vi "Compute N-Exp Fit Optimal Offset.vi"(7 "Fit Control Data in":T8, 8 "Error In":errorcluster, 9 "Offset Array":dbl[](array[numeric]), 11 "Fit Output in":T1[](array[typedef])) -> (0 "Error Out":errorcluster, 1 "C_00":dbl, 3 "Fit Output out":T1={"best nonlinear fit"=[], "best fit parameters"=[], "R^2"=0.0, "RMSE"=0.0, "error out"={"status"=FALSE, "code"=0, "source"=""}, "Fitting Method"=enum."Least Square", "number of function calls"=0, "number of iterations"=0, "covariance"=[], "Chi 2"=0.0, "DOF"=0, "Fit Convergence Criterion"=enum."Continue", "Fitting Algorithm"=enum."Levenberg-Marquardt", "Weighted Fit"=enum."Unweighted", "Gradient"=0.0, "|Delta Chi 2|"=0.0, "|Delta Chi 2|/Chi 2"=0.0, "Max |Delta a| /|a|"=0.0, "Lambda"=-1.0, "RSS"=0.0, "AIC"=0.0, "BIC"=0.0, "Max number of function calls"=0, "Max number of iterations"=0, "IRF"={"X Array"=[], "Y Array"=[]}, "IRF Normalization Factor"=0.0, "Decay Normalization Factor"=0.0, "Number of offset fits"=0, "Weighted Chi2"=-1.0, "Unweighted Chi2"=-1.0}, 5 "Fit Control Data out":T8)   [LabVIEW 2021, in "Fits.lvlib"]
doc: "If more than 2 offsets have been tried, fits a parabola through the Chi^2 values to find the minimum location. and returns the curvatue C_00 used to computed the offset uncertainty.\nOtherwise, use the result with the smallest Chi^2."
uses:
  Fits.lvlib
  Non-linear Fit Output v4.ctl
  Nonlinear Fit Method.ctl
  <vilib>/Analysis/Matrix/Datatypes/RealMatrix.ctl
  Convergence Criteria.ctl
  Non-linear Fitting Algorithm.ctl
  IRF(X)PSED/Fit Weights Type v2.ctl
  Graphs/XY Graph/XY Graph Plot Data.ctl
  Decay Convolution/Fit Control Data v2.ctl
  IRF(X)PSED/Decay Fit Parameters In List.ctl
  Decay Convolution/Decay Model.ctl
  <vilib>/Analysis/Matrix/NI_Matrix.lvlib
  Graphs/XY Graph/XY Graph Add-Ons.lvlib
panel:
  out "~t_0":dbl
  out "Chi^2":dbl
  out "t_0":dbl
  out "XY Graph":T11(graph)
  # "see the AlliGator License on the block diagram (Ctrl+E or Window:Show Block Diagram)"
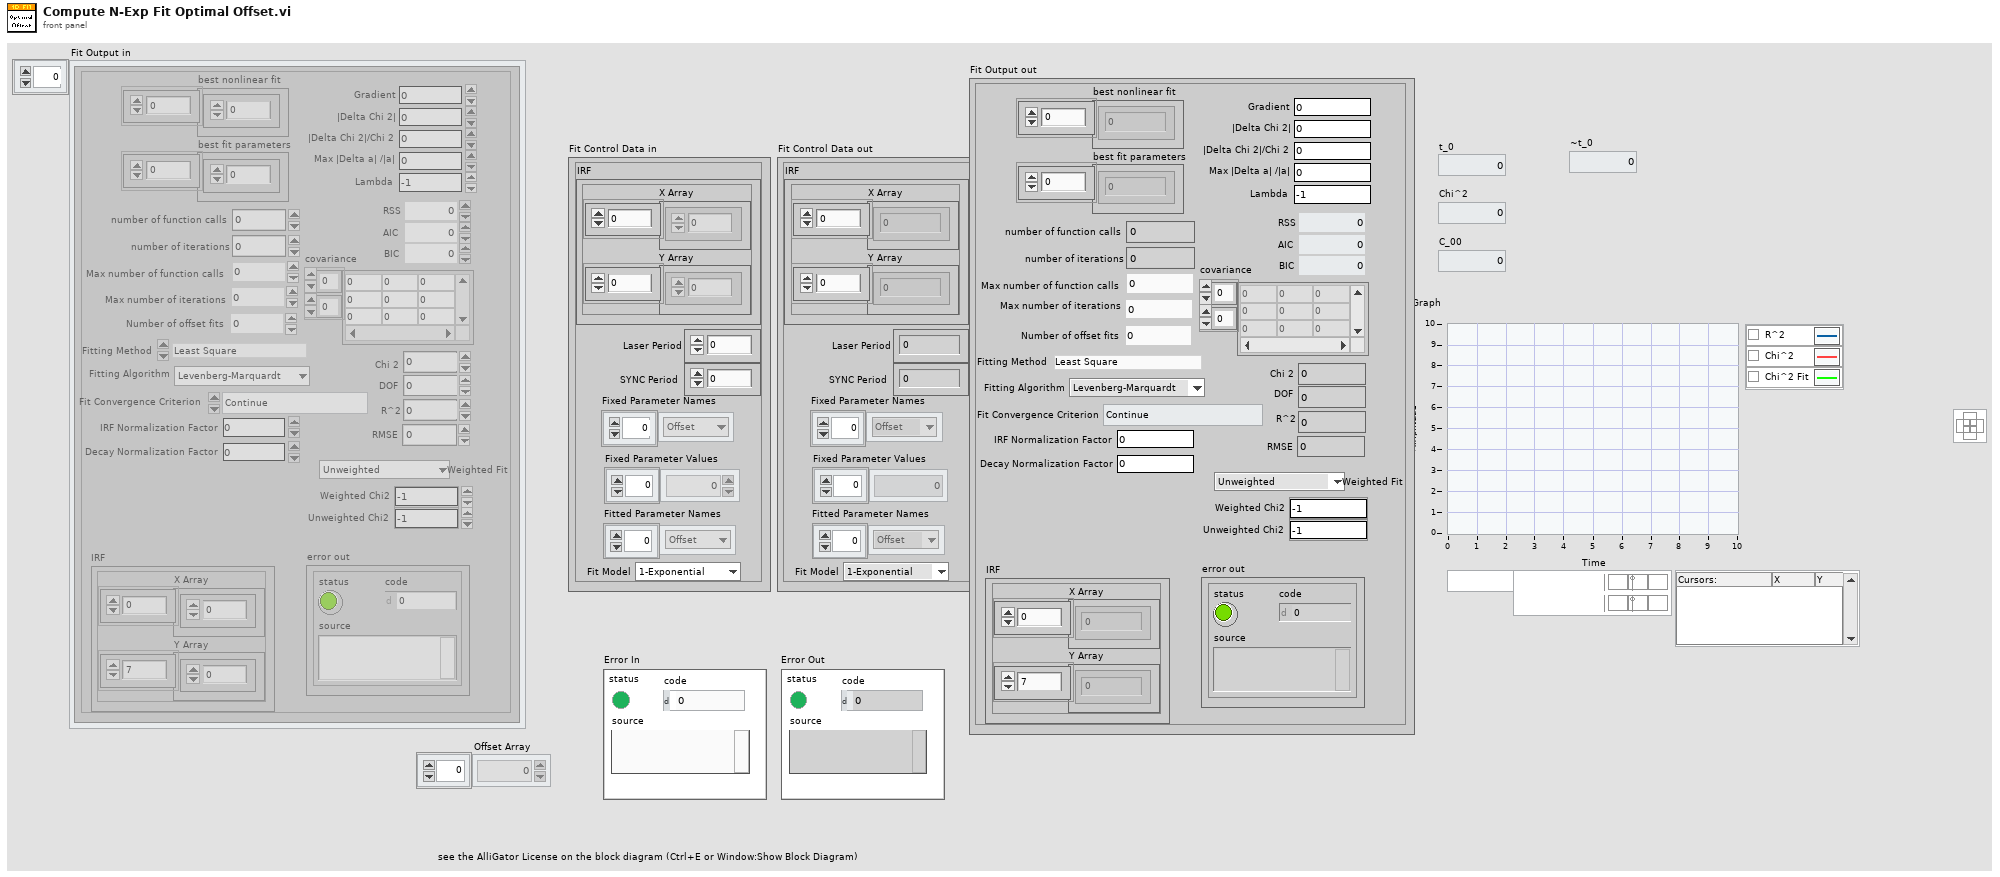
[diagram p1: front panel]
types:
  T1 = typedef "Fits.lvlib/Non-linear Fit Output v4.ctl" = cluster{"best nonlinear fit":dbl[], "best fit parameters":dbl[], "R^2":dbl, "RMSE":dbl, "error out":errorcluster, "Fitting Method":T2, "number of function calls":i32, "number of iterations":i32, "covariance":T3, "Chi 2":dbl, "DOF":i32, "Fit Convergence Criterion":T4, "Fitting Algorithm":T5, "Weighted Fit":T6, "Gradient":dbl, "|Delta Chi 2|":dbl, "|Delta Chi 2|/Chi 2":dbl, "Max |Delta a| /|a|":dbl, "Lambda":dbl, "RSS":dbl, "AIC":dbl, "BIC":dbl, "Max number of function calls":i32, "Max number of iterations":i32, "IRF":T7, "IRF Normalization Factor":dbl, "Decay Normalization Factor":dbl, "Number of offset fits":i32, "Weighted Chi2":dbl, "Unweighted Chi2":dbl}
  T2 = typedef "Fits.lvlib/Nonlinear Fit Method.ctl" = enum16{"Least Square", "Least Absolute Residual", "Bisquare", "MLE"}
  T3 = typedef "NI_Matrix.lvlib/RealMatrix.ctl" = dbl[][]
  T4 = typedef "Fits.lvlib/Convergence Criteria.ctl" = enum16{"Continue", "Tolerances Exceeded", "Max Time Exceeded", "Max Iterations Exceeded", "Max Function Evaluations Exceeded", "Scale Range Exceeded"}
  T5 = typedef "Fits.lvlib/Non-linear Fitting Algorithm.ctl" = enum16{"Levenberg-Marquardt", "Trust-Region Dogleg"}
  T6 = typedef "Fits.lvlib/Fit Weights Type v2.ctl" = enum16{"Unweighted", "1/Variance (Neyman)", "1/Variance (Pearson)", "Best of All"}
  T7 = typedef "XY Graph Add-Ons.lvlib/XY Graph Plot Data.ctl" = cluster{"X Array":dbl[], "Y Array":dbl[]}
  T8 = typedef "Fits.lvlib/Fit Control Data v2.ctl" = cluster{"IRF":T7, "Laser Period":dbl, "SYNC Period":dbl, "Fixed Parameter Names":T9[], "Fixed Parameter Values":dbl[], "Fitted Parameter Names":T9[], "Fit Model":T10}
  T9 = typedef "Fits.lvlib/Decay Fit Parameters In List.ctl" = enum16{"Offset", "Baseline", "A_1", "tau_1", "A_2", "tau_2"}
  T10 = typedef "Fits.lvlib/Decay Model.ctl" = enum16{"1-Exponential", "2-Exponentials"}
  T11 = cluster{"Offset Array":dbl[], "Best Polynomial Fit":dbl[]}[]
  T12 = cluster{"Offset Array used for Fit":dbl[], "Best Polynomial Fit":dbl[]}
  T13 = cluster{"Offset Array used for Fit":dbl[], "Best Polynomial Fit":dbl[]}[]
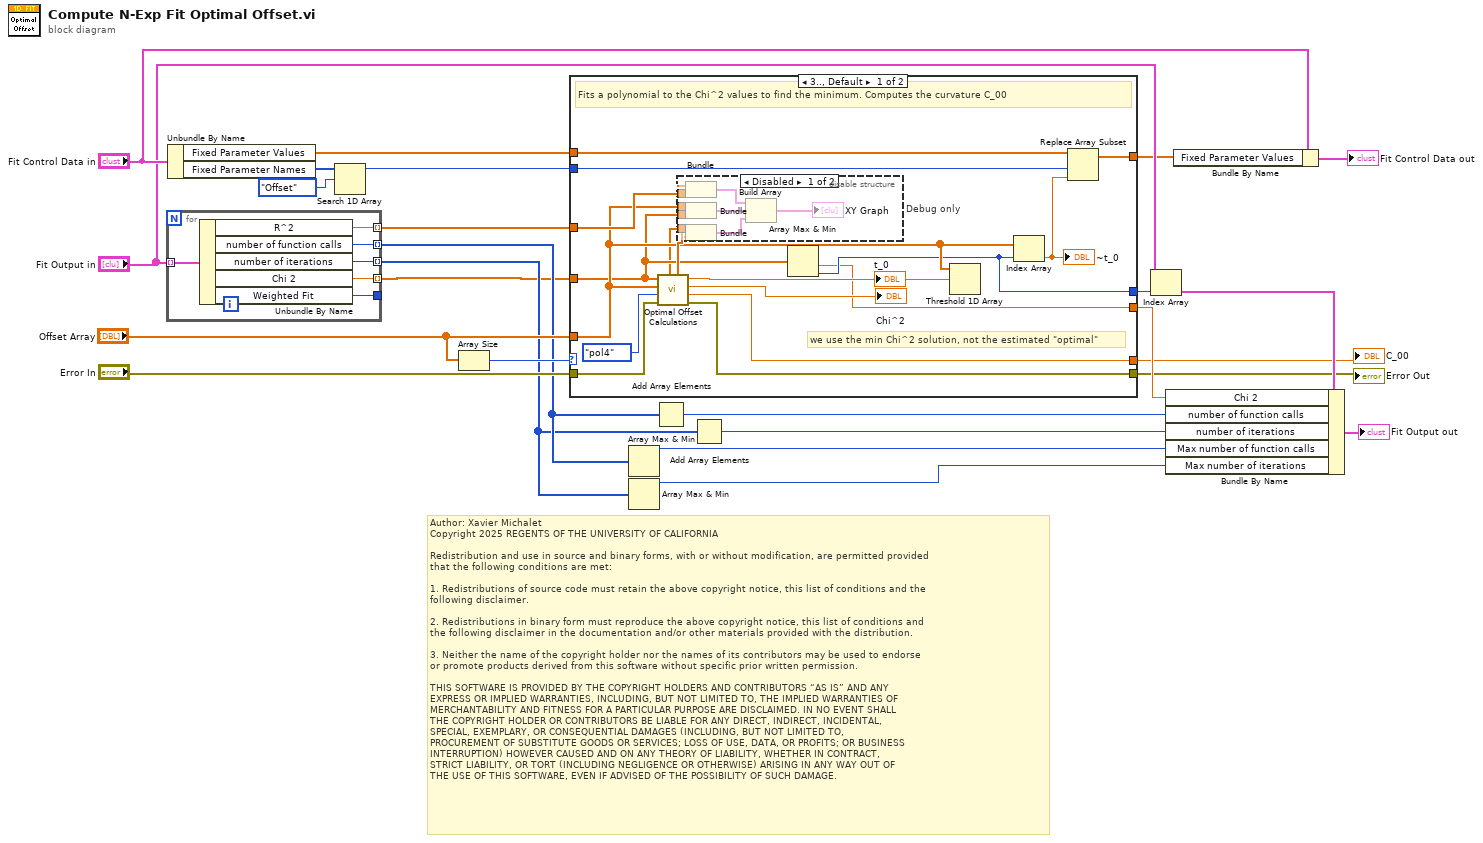
[diagram p0: block diagram]
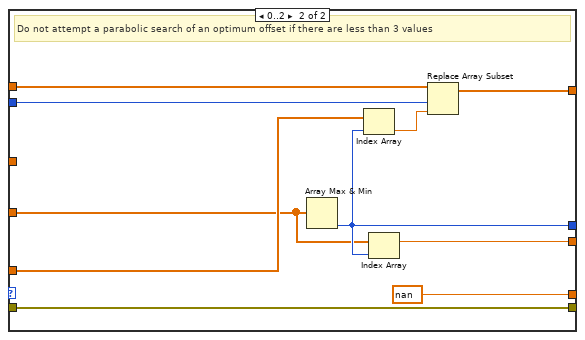
[diagram p3: hidden frame]
diagram:
  # "Author: Xavier Michalet\nCopyright 2025 REGENTS OF THE UNIVERSITY OF CALIFORNIA\n\nRedistribution and use in source and binary forms, with or without modification, are permitted provided\nthat the following conditions are met:\n\n1. Redistributions of source code must retain the above copyright notice, this list of conditions and the\nfollowing disclaimer.\n\n2. Redistributions in binary form must reproduce the above copyright notice, this list of conditions and\nthe following disclaimer in the documentation and/or other materials provided with the distribution.\n\n3. Neither the name of the copyright holder nor the names of its contributors may be used to endorse \nor promote products derived from this software without specific prior written permission.\n\nTHIS SOFTWARE IS PROVIDED BY THE COPYRIGHT HOLDERS AND CONTRIBUTORS “AS IS” AND ANY \nEXPRESS OR IMPLIED WARRANTIES, INCLUDING, BUT NOT LIMITED TO, THE IMPLIED WARRANTIES OF\nMERCHANTABILITY AND FITNESS FOR A PARTICULAR PURPOSE ARE DISCLAIMED. IN NO EVENT SHALL\nTHE COPYRIGHT HOLDER OR CONTRIBUTORS BE LIABLE FOR ANY DIRECT, INDIRECT, INCIDENTAL, \nSPECIAL, EXEMPLARY, OR CONSEQUENTIAL DAMAGES (INCLUDING, BUT NOT LIMITED TO, \nPROCUREMENT OF SUBSTITUTE GOODS OR SERVICES; LOSS OF USE, DATA, OR PROFITS; OR BUSINESS\nINTERRUPTION) HOWEVER CAUSED AND ON ANY THEORY OF LIABILITY, WHETHER IN CONTRACT, \nSTRICT LIABILITY, OR TORT (INCLUDING NEGLIGENCE OR OTHERWISE) ARISING IN ANY WAY OUT OF\nTHE USE OF THIS SOFTWARE, EVEN IF ADVISED OF THE POSSIBILITY OF SUCH DAMAGE."
  n1 = for {
    tunnel: "Fit Output in" -> [w31] mode=indexing
    tunnel: [w30] -> w1 mode=indexing
    tunnel: [w29] -> w5 mode=indexing
    tunnel: [w28] -> w3 mode=indexing
    tunnel: [w27] -> w8 mode=indexing
    tunnel: [w26] -> _
    n2 = Unbundle By Name(w31) -> ("R^2"=w27:dbl, "number of function calls"=w29:i32, "number of iterations"=w28:i32, "Chi 2"=w30:dbl, "Weighted Fit"=w26:T6)
  }
  n3 = Unbundle By Name("Fit Control Data in") -> ("Fixed Parameter Values"=w18:dbl[], "Fixed Parameter Names"=w20:T9[])
  n4 = Search 1D Array(1D array=w20, element=Decay_Fit_Parameters_In_List."Offset") -> (index of element=w17:i32)  [unwired: 1 in]
  n5 = Array Size(array="Offset Array") -> (size(s)=w10:i32)
  n6 = case shown="3.., Default" w10 {
    tunnel: "Offset Array" -> [w39 w67]
    tunnel: w1 -> [w34 w60]
    tunnel: w18 -> [w37 w66]
    tunnel: w17 -> [w38 w65]
    tunnel: [w48 w64] -> w16
    tunnel: [w32 w62] -> w14
    tunnel: [w36 w61] -> w11
    tunnel: [w44 nan ("C00")] -> w9
    tunnel: w8 -> [w47 _]
    tunnel: "Error In" -> [w46 w58]
    tunnel: [w45 w58] -> w6
    frame 3.., Default {
      # "we use the min Chi^2 solution, not the estimated \"optimal\""
      # "Fits a polynomial to the Chi^2 values to find the minimum. Computes the curvature C_00"
      n7 = call "Optimal Offset Calculations.vi"("Error In"=w46, "Polynomial"=enum16{"pol2", "pol4"}."pol4", "Offset Array"=w39, "Chi^2 Array"=w34) -> ("Error Out"=w45:errorcluster, "C00"=w44:dbl, "Chi^2"=→"Chi^2":dbl, "t0"=w42:dbl, "Best Polynomial Fit"=w43:dbl[], "Offset Array used for Fit"=w33:dbl[])  [unwired: 2 in]
      "t_0" <- w42
      n8 = disable-structure "Debug only" shown="Disabled" {
        disable-tunnel: w47 -> [w54 _]
        disable-tunnel: w43 -> [w52 _]
        disable-tunnel: w39 -> [w51 _]
        disable-tunnel: w34 -> [w50 _]
        disable-tunnel: w33 -> [w49 _]
        frame Disabled {
          n9 = Bundle("Offset Array"=w51, w54) -> (w53:cluster{"Offset Array":dbl[], dbl[]})  [unwired: 1 in]
          n10 = Bundle("Offset Array"=w51, w50) -> (w57:cluster{"Offset Array":dbl[], dbl[]})  [unwired: 1 in]
          n11 = Bundle("Offset Array used for Fit"=w49, "Best Polynomial Fit"=w52) -> (w56:T12)  [unwired: 1 in]
          n12 = Build Array(w53, w57, w56) -> (→"XY Graph":T13)
        }
        frame Enabled {
        }
      }
      n13 = Array Max & Min(array=w34) -> (min value=w32:dbl, min index (indices)=w36:i32)  [unwired: 2 out]
      n14 = Threshold 1D Array(2:w42, 3:w39) -> ()  [unwired: 1 in, 1 out]
      n15 = Index Array(array=w39, index=w36) -> (element=w35:dbl)
      "~t_0" <- w35
      n16 = Replace Array Subset(array=w37, new element=w35, index=w38) -> (w48:dbl[])
    }
    frame 0..2 {
      # "Do not attempt a parabolic search of an optimum offset if there are less than 3 values"
      n17 = Array Max & Min(array=w60) -> (min index (indices)=w61:i32)  [unwired: 3 out]
      n18 = Index Array(array=w67, index=w61) -> (element=w63:dbl)
      n19 = Index Array(array=w60, index=w61) -> (element=w62:dbl)
      n20 = Replace Array Subset(array=w66, new element=w63, index=w65) -> (w64:dbl[])
    }
  }
  "Error Out" <- w6
  "C_00" <- w9
  n21 = Array Max & Min(array=w5) -> (max value=w4:i32)  [unwired: 3 out]
  n22 = Array Max & Min(array=w3) -> (max value=w2:i32)  [unwired: 3 out]
  n23 = Add Array Elements(numeric array=w5) -> (sum=w13:i32)
  n24 = Add Array Elements(numeric array=w3) -> (sum=w12:i32)
  n25 = Index Array(array="Fit Output in", index=w11) -> (element=w15:T1)
  n26 = Bundle By Name(cluster=w15, "Chi 2"=w14, "number of function calls"=w13, "number of iterations"=w12, "Max number of function calls"=w4, "Max number of iterations"=w2) -> (→"Fit Output out":T1)
  n27 = Bundle By Name(cluster="Fit Control Data in", "Fixed Parameter Values"=w16) -> (→"Fit Control Data out":T8)
